vi "layoutVirtual.vi"(0 "reference":refnum<class "Graph.lvclass">, 1 "graphics":refnum<class "Graphics.lvclass">, 2 "grid":refnum<class "Grid.lvclass">, 5 "error in (no error)":errorcluster) -> (14 "reference out":refnum<class "Graph.lvclass">, 19 "error out":errorcluster)   [LabVIEW 2014, in "Graph.lvclass"]
doc: "public void layout()"
uses:
  <resource>/Framework/Providers/Open_GDS/UML/Graph_class/Graph.lvclass
  <resource>/Framework/Providers/Open_GDS/UML/Grid_class/Grid.lvclass
  <resource>/Framework/Providers/Open_GDS/UML/Graphics_class/Graphics.lvclass
  <resource>/Framework/Providers/Open_GDS/UML/AbstractNode_class/AbstractNode.lvclass
  <resource>/Framework/Providers/Open_GDS/UML/AbstractEdge_class/AbstractEdge.lvclass
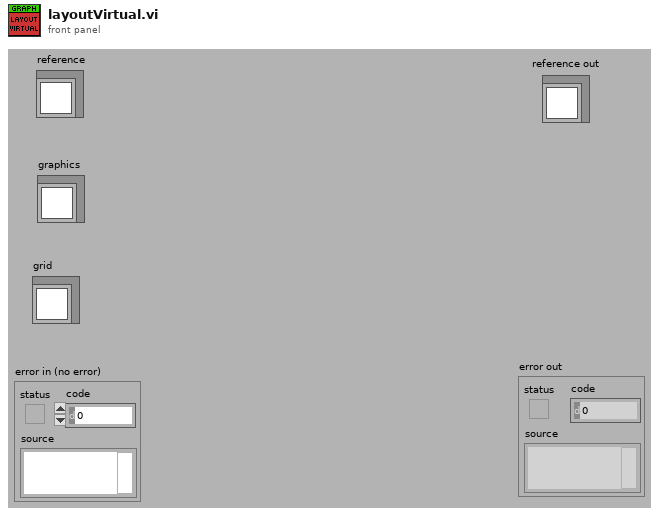
[diagram p1: front panel]
types:
  T1 = typedef "Graph.lvclass/ObjectAttributes.ctl" = cluster{"nodes":refnum<class "AbstractNode.lvclass">[], "edges":refnum<class "AbstractEdge.lvclass">[], "nodesToBeRemoved":refnum<class "AbstractNode.lvclass">[], "edgesToBeRemoved":refnum<class "AbstractEdge.lvclass">[], "needsLayout":bool, "LayoutNodes":refnum<class "AbstractNode.lvclass">[]}
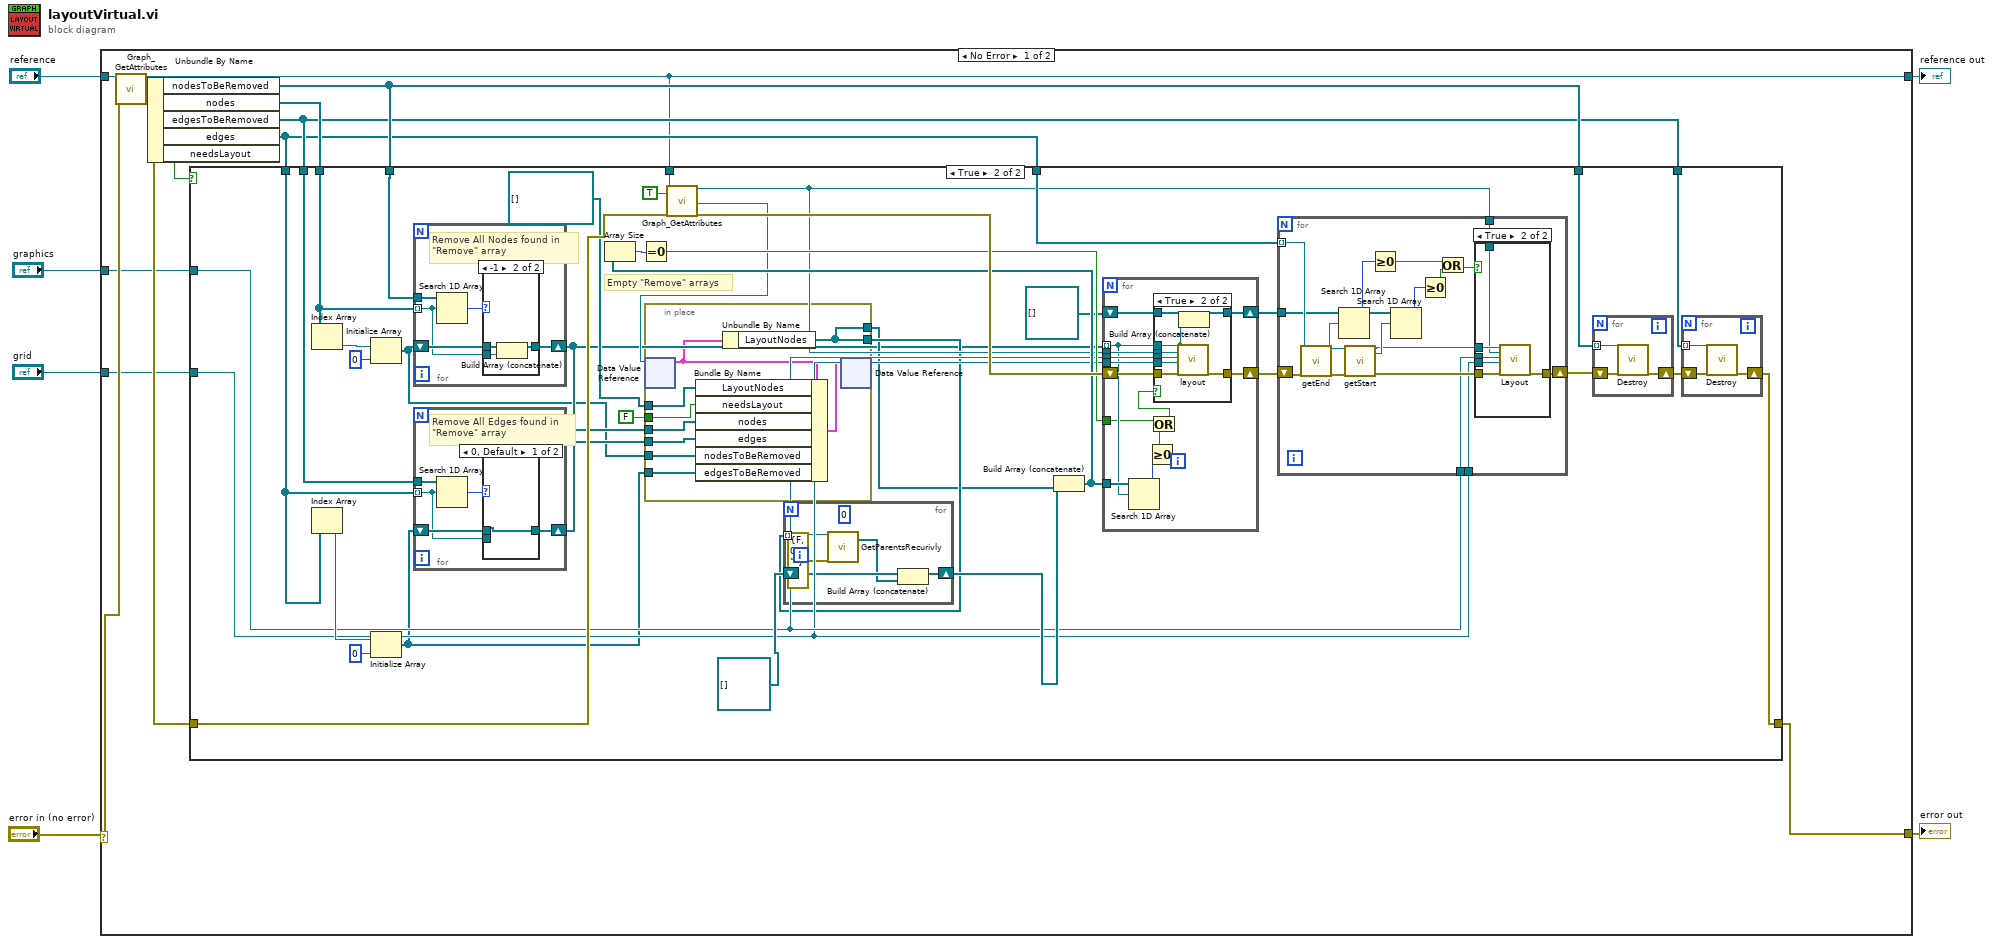
[diagram p0: block diagram]
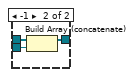
[diagram p5: hidden frame]
diagram:
  n1 = case shown="No Error" "error in (no error)" {
    selector: "error in (no error)" -> [w15 w145]
    tunnel: "reference" -> [w19 w146]
    tunnel: [w18 w145] -> w5
    tunnel: [w8 w146] -> w4
    tunnel: "graphics" -> [w13 _]
    tunnel: "grid" -> [w12 _]
    frame No Error {
      n2 = call <resource>:"Graph_GetAttributes.vi"("reference in"=w19, "error in (no error)"=w15) -> ("reference out"=w8:refnum<class "Graph.lvclass">, "Data"=w7:T1, "error out"=w17:errorcluster)  [unwired: 1 in, 14 out]
      n3 = Unbundle By Name(w7) -> ("nodesToBeRemoved"=w11:refnum<class "AbstractNode.lvclass">[], "nodes"=w14:refnum<class "AbstractNode.lvclass">[], "edgesToBeRemoved"=w10:refnum<class "AbstractEdge.lvclass">[], "edges"=w9:refnum<class "AbstractEdge.lvclass">[], "needsLayout"=w16:bool)
      n4 = case shown="True" w16 {
        tunnel: w17 -> [w20 w49]
        tunnel: [w20 w44] -> w18
        tunnel: w11 -> [_ w53]
        tunnel: w14 -> [_ w54]
        tunnel: w10 -> [_ w51]
        tunnel: w9 -> [_ w52]
        tunnel: w8 -> [_ w50]
        tunnel: w13 -> [_ w35]
        tunnel: w12 -> [_ w34]
        tunnel: w11 -> [_ w47]
        tunnel: w10 -> [_ w45]
        tunnel: w9 -> [_ w37]
        frame False {
        }
        frame True {
          # "Empty \"Remove\" arrays"
          n5 = Index Array(array=w54) -> (element=w58:refnum<class "AbstractNode.lvclass">)  [unwired: 1 in]
          n6 = Index Array(array=w52) -> (element=w55:refnum<class "AbstractEdge.lvclass">)  [unwired: 1 in]
          n7 = Initialize Array(w58, 0 ("dimension size")) -> (w22:refnum<class "AbstractNode.lvclass">[])
          n8 = Initialize Array(w55, 0 ("dimension size")) -> (w21:refnum<class "AbstractEdge.lvclass">[])
          n9 = for {
            tunnel: w54 -> [w137] mode=indexing
            tunnel: w53 -> [w140]
            shift-right: [w136] -> w24
            shift-left: w22 -> [w138]
            # "Remove All Nodes found in\n\"Remove\" array"
            n10 = Search 1D Array(1D array=w140, element=w137) -> (index of element=w139:i32)  [unwired: 1 out]
            n11 = case shown="-1" w139 {
              tunnel: w138 -> [w141 w144]
              tunnel: w137 -> [_ w143]
              tunnel: [w141 w142] -> w136
              frame 0, Default {
              }
              frame -1 {
                n12 = Build Array (concatenate)(w144, w143) -> (w142:refnum<class "AbstractNode.lvclass">[])
              }
            }
          }
          n13 = for {
            tunnel: w52 -> [w128] mode=indexing
            tunnel: w51 -> [w131]
            shift-right: [w127] -> w23
            shift-left: w21 -> [w129]
            # "Remove All Edges found in\n\"Remove\" array"
            n14 = Search 1D Array(1D array=w131, element=w128) -> (index of element=w130:i32)  [unwired: 1 out]
            n15 = case shown="0, Default" w130 {
              tunnel: w129 -> [w132 w135]
              tunnel: w128 -> [_ w134]
              tunnel: [w132 w133] -> w127
              frame 0, Default {
              }
              frame -1 {
                n16 = Build Array (concatenate)(w135, w134) -> (w133:refnum<class "AbstractEdge.lvclass">[])
              }
            }
          }
          n17 = call <resource>:"Graph_GetAttributes.vi"("reference in"=w50, "OnlyGetDvrReference(False)"=TRUE, "error in (no error)"=w49) -> ("reference out"=w33:refnum<class "Graph.lvclass">, "DataRef"=w29:refnum<data-value>, "error out"=w48:errorcluster)  [unwired: 13 in, 1 out]
          n18 = in-place {
            in-place-border: [w66] -> w28
            in-place-border: [w66] -> w27
            in-place-border: refnum<class "AbstractNode.lvclass">[] [] ("LayoutNodes") -> [w65]
            in-place-border: FALSE ("needsLayout") -> [w64]
            in-place-border: w24 -> [w63]
            in-place-border: w23 -> [w62]
            in-place-border: w22 -> [w61]
            in-place-border: w21 -> [w60]
            n19 = in-place-dvr #1(w29) -> (w67:T1)  [unwired: 1 out]
            n20 = Bundle By Name(cluster=w67, "LayoutNodes"=w65, "needsLayout"=w64, "nodes"=w63, "edges"=w62, "nodesToBeRemoved"=w61, "edgesToBeRemoved"=w60) -> (w59:T1)
            n21 = Unbundle By Name(w67) -> ("LayoutNodes"=w66:refnum<class "AbstractNode.lvclass">[])
            n22 = in-place-dvr #1(w59) -> ()  [unwired: 2 out]
          }
          n23 = for {
            tunnel: w28 -> [w95] mode=indexing
            shift-right: [w96] -> w39
            shift-left: refnum<class "AbstractNode.lvclass">[] [] ("LayoutNodes") -> [w97]
            (unwired) 0
            n24 = call-dynamic "GetParentsRecurivly.vi"("reference"=w95, "error in (no error)"=errorcluster {"status"=FALSE, "code"=0, "source"=""}) -> ("Parents"=w94:refnum<class "AbstractNode.lvclass">[])  [unwired: 15 in, 2 out]
            n25 = Build Array (concatenate)(w97, w94) -> (w96:refnum<class "AbstractNode.lvclass">[])
          }
          n26 = Build Array (concatenate)(w39, w27) -> (w40:refnum<class "AbstractNode.lvclass">[])
          n27 = Array Size(array=w40) -> (size(s)=w43:i32)
          n28 = Equal To 0?(x=w43) -> (x = 0?=w42:bool)
          n29 = for {
            tunnel: w24 -> [w110] mode=indexing
            tunnel: w33 -> [w116]
            tunnel: w35 -> [w115]
            tunnel: w34 -> [w114]
            shift-right: [w112] -> w36
            shift-left: w48 -> [w113]
            tunnel: w40 -> [w111]
            tunnel: w42 -> [w108]
            shift-right: [w105] -> w32
            shift-left: refnum<class "AbstractNode.lvclass">[] [] ("LayoutNodes") -> [w104]
            n30 = Search 1D Array(1D array=w111, element=w110) -> (index of element=w109:i32)  [unwired: 1 out]
            n31 = Greater Or Equal To 0?(x=w109) -> (x >= 0?=w107:bool)
            n32 = Or(x=w108, y=w107) -> (x .or. y?=w106:bool)
            n33 = case shown="True" w106 {
              tunnel: w116 -> [_ w126]
              tunnel: w115 -> [_ w125]
              tunnel: w114 -> [_ w124]
              tunnel: w113 -> [w118 w123]
              tunnel: [w118 w122] -> w112
              tunnel: w110 -> [_ w120]
              tunnel: w104 -> [w117 w121]
              tunnel: [w117 w119] -> w105
              frame False {
              }
              frame True {
                n34 = call-dynamic "layout.vi"("reference"=w120, "graph"=w126, "graphics"=w125, "grid"=w124, "error in (no error)"=w123) -> ("error out"=w122:errorcluster)  [unwired: 13 in, 1 out]
                n35 = Build Array (concatenate)(w121, w120) -> (w119:refnum<class "AbstractNode.lvclass">[])
              }
            }
          }
          n36 = for {
            tunnel: w37 -> [w82] mode=indexing
            shift-right: [w74] -> w31
            shift-left: w36 -> [w85]
            tunnel: w32 -> [w80]
            tunnel: w35 -> [w70]
            tunnel: w33 -> [w69]
            tunnel: w34 -> [w68]
            n37 = call-dynamic "getEnd.vi"("reference"=w82, "error in (no error)"=w85) -> ("reference out"=w84:refnum<class "AbstractEdge.lvclass">, "endNode"=w81:refnum<class "AbstractNode.lvclass">, "error out"=w83:errorcluster)  [unwired: 14 in, 1 out]
            n38 = Search 1D Array(1D array=w80, element=w81) -> (index of element=w78:i32)  [unwired: 1 out]
            n39 = call-dynamic "getStart.vi"("reference"=w84, "error in (no error)"=w83) -> ("reference out"=w71:refnum<class "AbstractEdge.lvclass">, "startNode"=w79:refnum<class "AbstractNode.lvclass">, "error out"=w73:errorcluster)  [unwired: 14 in, 1 out]
            n40 = Greater Or Equal To 0?(x=w78) -> (x >= 0?=w75:bool)
            n41 = Search 1D Array(1D array=w80, element=w79) -> (index of element=w77:i32)  [unwired: 1 out]
            n42 = Greater Or Equal To 0?(x=w77) -> (x >= 0?=w76:bool)
            n43 = Or(x=w75, y=w76) -> (x .or. y?=w72:bool)
            n44 = case shown="True" w72 {
              tunnel: [w86 w92] -> w74
              tunnel: w73 -> [w86 w91]
              tunnel: w71 -> [_ w90]
              tunnel: w70 -> [_ w89]
              tunnel: w69 -> [_ w88]
              tunnel: w68 -> [_ w87]
              frame False {
              }
              frame True {
                n45 = call-dynamic "Layout.vi"("reference"=w90, "graph"=w88, "graphics"=w89, "grid"=w87, "error in (no error)"=w91) -> ("error out"=w92:errorcluster)  [unwired: 13 in, 1 out]
              }
            }
          }
          n46 = for {
            tunnel: w47 -> [w103] mode=indexing
            shift-right: [w101] -> w46
            shift-left: w31 -> [w102]
            n47 = call-dynamic "Destroy.vi"("reference"=w103, "error in (no error)"=w102) -> ("error out"=w101:errorcluster)  [unwired: 16 in, 1 out]
          }
          n48 = for {
            tunnel: w45 -> [w100] mode=indexing
            shift-right: [w98] -> w44
            shift-left: w46 -> [w99]
            n49 = call-dynamic "Destroy.vi"("reference"=w100, "error in (no error)"=w99) -> ("error out"=w98:errorcluster)  [unwired: 17 in]
          }
        }
      }
    }
    frame Error {
    }
  }
  "reference out" <- w4
  "error out" <- w5
